vi "3D Contour Graph.vi"() -> ()   [LabVIEW 2023]
doc: "This VI shows how to use the 3D Contour Plot."
uses:
  <vilib>/Math Plots/3D Math Plots/3D Contour/3D Contour XCtrl/3D Contour.xctl
  <vilib>/Math Plots/3D Math Plots/3D Contour/3D Contour Datatype/Public/Plot Helper (Vector).vi
  <vilib>/Math Plots/3D Math Plots/3D Contour/3D Contour Datatype/3D Contour Datatype.lvclass
panel:
  out "3D Contour":refnum<class "3D Plot Datatype.lvclass">[](xcontrol)
  # "Overview: Demonstrates the Contour indicator from the Graph > 3D Graph palette.\nRequirements: LabVIEW Full Development System\nInstructions:\nRun the VI."
  # "Try the following operations on the graph:\n\n1. Click and drag the mouse within the graph to change the view direction.\n2. Press the Shift key and drag the mouse up to zoom in.\n3. Press the Shift key and drag the mouse down to zoom out.\n4. Right-click the graph and choose 3D Plot Properties to configure various properties related to the graph's appearance.\n5. Right-click the graph and select Export Image >Export to File."
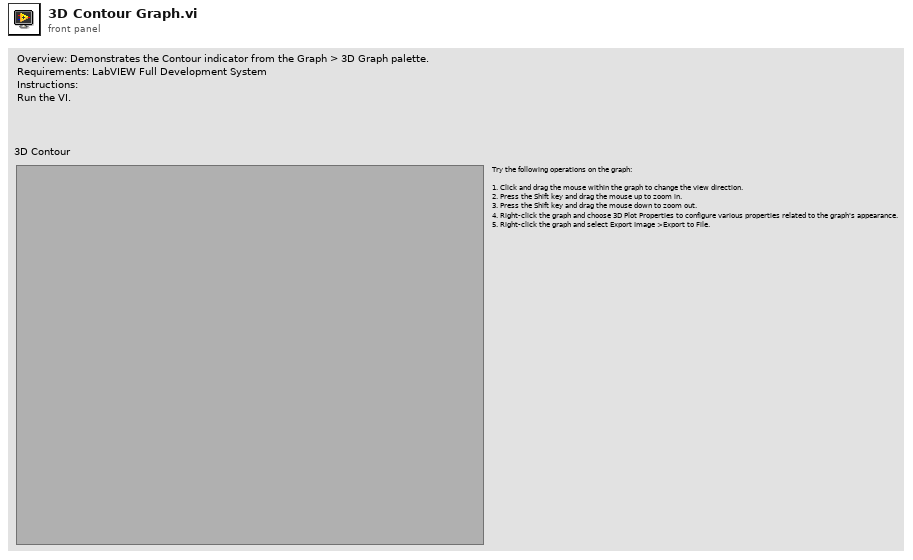
[diagram p1: front panel]
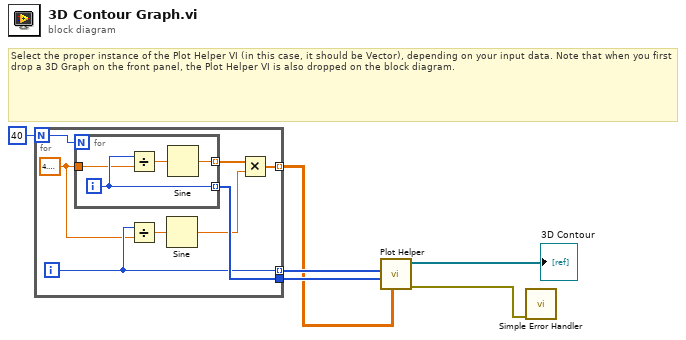
[diagram p0: block diagram]
diagram:
  # "Select the proper instance of the Plot Helper VI (in this case, it should be Vector), depending on your input data. Note that when you first drop a 3D Graph on the front panel, the Plot Helper VI is also dropped on the block diagram."
  n1 = for {
    N: 40 ("X input length") -> [w8]
    tunnel: [w14] -> w4
    tunnel: [w10] -> w3 mode=indexing
    tunnel: [w9] -> w5 mode=indexing
    i -> [w9]
    w7 = sgl 4.2 ("y")
    n2 = for {
      N: w8 -> [_]
      tunnel: [w17] -> w12 mode=indexing
      tunnel: [w16] -> w14 mode=indexing
      tunnel: w7 -> [w15]
      i -> [w16]
      n3 = Divide(x=w16, y=w15) -> (x/y=w18:sgl)
      n4 = Sine(x=w18) -> (sin(x)=w17:sgl)
    }
    n5 = Divide(x=w9, y=w7) -> (x/y=w13:sgl)
    n6 = Sine(x=w13) -> (sin(x)=w11:sgl)
    n7 = Multiply(x=w12, y=w11) -> (x*y=w10:sgl[])
  }
  n8 = call-poly <vilib>:"Plot Helper.vi"("z matrix"=w3, "y vector"=w4, "x vector"=w5) -> ("error out"=w1:errorcluster, "3D Plot lvclass Array out"=→"3D Contour":refnum<class "3D Plot Datatype.lvclass">[])  [unwired: 3 in, 4 out]
  n9 = call <vilib>:"Simple Error Handler.vi"("error in (no error)"=w1) -> ()  [unwired: 4 in, 5 out]
